vi "Noise Figure Display Setup.vi"(0 "VISA resource name":refnum<visa-resource-name>, 5 "Measurement Type (0: Gain)":u16(ring) items=["Gain", "Noise Figure", "Noise Factor", "Cold Power Density", "Hot Power Density", "Effective Temperature", "Tcold", "Y Factor"], 7 "Y-Axis Scale Per Division (5 dB)":dbl=5.0 format="%^#_6g", 9 "Y-Axis Reference Level (15 dB)":dbl=15.0 format="%^#_6g", 11 "error in (no error)":errorcluster, 12 "Upper Display Mode (0: Gain)":u16(ring) items=["Gain", "Noise Figure", "Noise Factor", "Cold Power Density", "Hot Power Density", "Effective Temperature", "Y Factor"], 13 "Lower Display Mode (1: Noise Figure)":u16(ring)=1 items=["Gain", "Noise Figure", "Noise Factor", "Cold Power Density", "Hot Power Density", "Effective Temperature", "Y Factor"]) -> (4 "VISA resource name out":refnum<visa-resource-name>, 15 "error out":errorcluster)   [LabVIEW 2014, in "Agilent ESA PSA Series.lvlib"]
doc: "Configures the Noise Figure measurement display of the Noise Figure personality.\n\n<B>Note:</B>\n\nThis VI is only valid in Noise Figure personality. Use <B>Switch Personality</B> VI to switch to Noise Figure before calling this VI."
uses:
  Agilent ESA PSA Series.lvlib
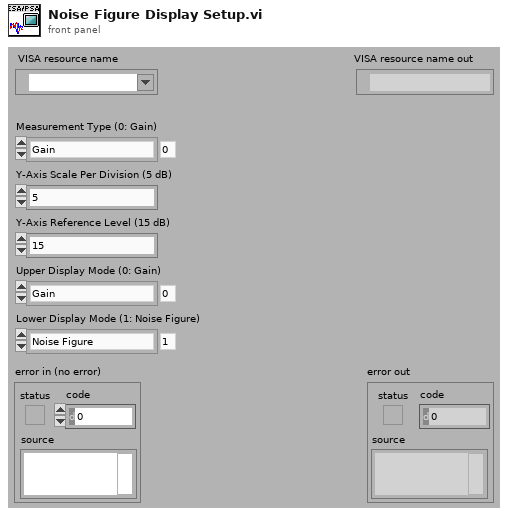
[diagram p1: front panel]
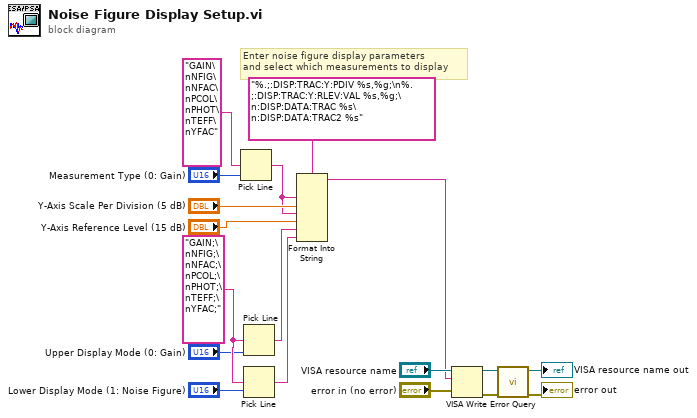
[diagram p0: block diagram]
diagram:
  w7 = "GAIN;\nNFIG;\nNFAC;\nPCOL;\nPHOT;\nTEFF;\nYFAC;" ("multi-line string")
  # "Enter noise figure display parameters\nand select which measurements to display"
  n1 = Pick Line(multi-line string="GAIN\nNFIG\nNFAC\nPCOL\nPHOT\nTEFF\nYFAC", line index="Measurement Type (0: Gain)") -> (output string=w6:string)  [unwired: 1 in]
  n2 = Pick Line(multi-line string=w7, line index="Upper Display Mode (0: Gain)") -> (output string=w4:string)  [unwired: 1 in]
  n3 = Pick Line(multi-line string=w7, line index="Lower Display Mode (1: Noise Figure)") -> (output string=w3:string)  [unwired: 1 in]
  n4 = Format Into String(format string="%.;:DISP:TRAC:Y:PDIV %s,%g;\n%.;:DISP:TRAC:Y:RLEV:VAL %s,%g;\n:DISP:DATA:TRAC %s\n:DISP:DATA:TRAC2 %s", w6, "Y-Axis Scale Per Division (5 dB)", w6, "Y-Axis Reference Level (15 dB)", w4, w3) -> (resulting string=w5:string)  [unwired: 2 in, 1 out]
  n5 = VISA Write(VISA resource name="VISA resource name", write buffer=w5, error in (no error)="error in (no error)") -> (VISA resource name out=w16:refnum<visa-resource-name>, error out=w15:errorcluster)  [unwired: 1 out]
  n6 = call "Error Query.vi"("error in (no error)"=w15, "VISA resource name"=w16) -> ("error out"=→"error out":errorcluster, "VISA resource name out"=→"VISA resource name out":refnum<visa-resource-name>)  [unwired: 6 in, 2 out]
